vi "Convert Configuration to Channels.vi"(8 "error in":errorcluster, 11 "_9226 Config Data":T3={"Conversion Time"=0, "Degree Range"=[], "RTD_Type"=[1], "RTD_A"=[], "RTD_B"=[], "RTD_C"=[], "RTD_Ro"=[]} {"Conversion Time" items=["200 ms", "2.5 ms"]; "Degree Range" items=["Raw Ohms", "Degrees Kelvin", "Degrees Celsius", "Degrees Fahrenheit", "Degrees Rankine"]; "RTD_Type" items=["TCR3851", "TCR3750", "TCR3916", "TCR3920", "TCR3911", "TCR3928", "Custom"]}) -> (0 "error out":errorcluster, 2 "Conversion Time":u32(ring) items=["200 ms", "2.5 ms"], 3 "Channels":T2(array[cluster]) {"RTD type" items=["User Defined"=0, "TCR3750"=2, "TCR3851"=7]})   [LabVIEW 2020, in "Modules.lvlib" / "9226.lvclass"]
uses:
  9226.lvclass
  Supported RTD Types.ctl
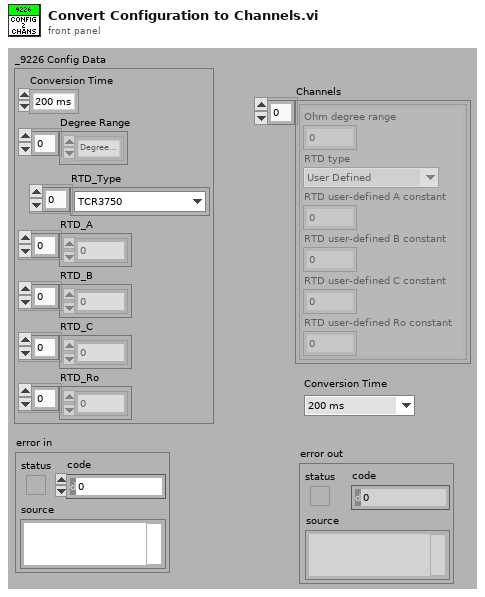
[diagram p1: front panel]
types:
  T1 = typedef "Modules.lvlib/9226.lvclass/Supported RTD Types.ctl" = u32
  T2 = cluster{"Ohm degree range":u32, "RTD type":T1, "RTD user-defined A constant":dbl, "RTD user-defined B constant":dbl, "RTD user-defined C constant":dbl, "RTD user-defined Ro constant":dbl}[]
  T3 = cluster{"Conversion Time":u32, "Degree Range":u32[], "RTD_Type":T1[], "RTD_A":dbl[], "RTD_B":dbl[], "RTD_C":dbl[], "RTD_Ro":dbl[]}
  T4 = cluster{"Ohm degree range":u32, "RTD type":T1, "RTD user-defined A constant":dbl, "RTD user-defined B constant":dbl, "RTD user-defined C constant":dbl, "RTD user-defined Ro constant":dbl}
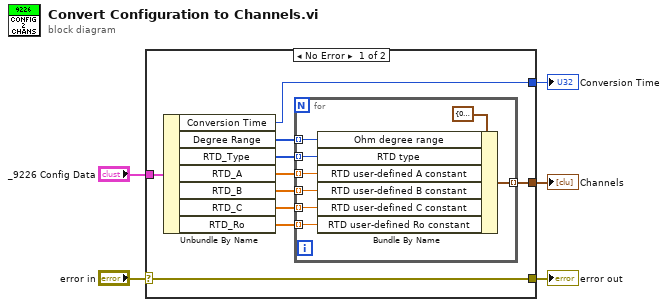
[diagram p0: block diagram]
diagram:
  n1 = case shown="No Error" "error in" {
    selector: "error in" -> [w15 w24]
    tunnel: [w15 w24] -> w4
    tunnel: "_9226 Config Data" -> [w14 _]
    tunnel: [w12 _] -> w2
    tunnel: [w6 _] -> w1
    frame No Error {
      n2 = Unbundle By Name(w14) -> ("Conversion Time"=w12:u32, "Degree Range"=w13:u32[], "RTD_Type"=w11:T1[], "RTD_A"=w10:dbl[], "RTD_B"=w9:dbl[], "RTD_C"=w8:dbl[], "RTD_Ro"=w7:dbl[])
      n3 = for {
        tunnel: w13 -> [w16] mode=indexing
        tunnel: w11 -> [w17] mode=indexing
        tunnel: w10 -> [w22] mode=indexing
        tunnel: w9 -> [w21] mode=indexing
        tunnel: w8 -> [w20] mode=indexing
        tunnel: w7 -> [w19] mode=indexing
        tunnel: [w18] -> w6 mode=indexing
        n4 = Bundle By Name(cluster=T4 {"Ohm degree range"=0, "RTD type"=0, "RTD user-defined A constant"=0.0, "RTD user-defined B constant"=0.0, "RTD user-defined C constant"=0.0, "RTD user-defined Ro constant"=0.0} ("Channel"), "Ohm degree range"=w16, "RTD type"=w17, "RTD user-defined A constant"=w22, "RTD user-defined B constant"=w21, "RTD user-defined C constant"=w20, "RTD user-defined Ro constant"=w19) -> (w18:T4)
      }
    }
    frame Error {
    }
  }
  "Channels" <- w1
  "error out" <- w4
  "Conversion Time" <- w2
